vi "NewBooks.vi"(2 "Username":string="ME 184", 3 "Dialog?":enum16{"No Dialog", "Dialog", "Overwrite"}(ring)=enum."Dialog", 4 "Remote Path":string="bookfiles/") -> ()   [LabVIEW 2012]
uses:
  <vilib>/RoboBookEngine/Server/HTTPServer/Server2_Globals.vi
  <userlib>/BotSpeak/Devices/EvalRIO/FTPCodes/FTPParameters.ctl
panel:
  out "Prefix":string="ME184"
  in  "Parameters":T1={"Book Folder Name"="", "Full file name"="", "Remote Path"="bookfiles/", "Shelf folder"=path "", "Existing books"=[], "Dialog?"=enum."No Dialog", "New Format?"=FALSE}
  out "status":string
  in  "Close":bool
  in  "Download":bool
  in  "Books":i32[](listbox)
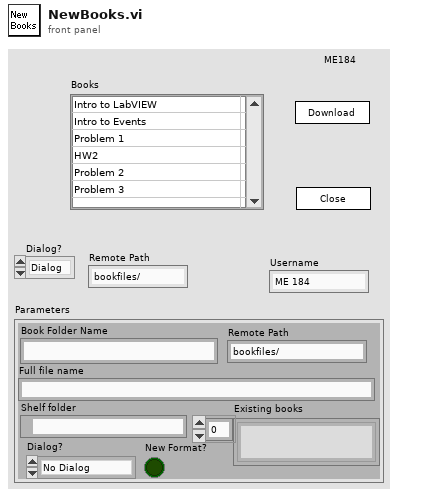
[diagram p1: front panel]
types:
  T1 = typedef "FTPParameters.ctl" = cluster{"Book Folder Name":string, "Full file name":string, "Remote Path":string, "Shelf folder":path, "Existing books":string[], "Dialog?":enum16{"No Dialog", "Dialog", "Overwrite"}, "New Format?":bool}
  T2 = typedef "PathsGlobal.ctl" = cluster{"Root":path, "Shelves":path, "Cmds":path, "Plugins":path}
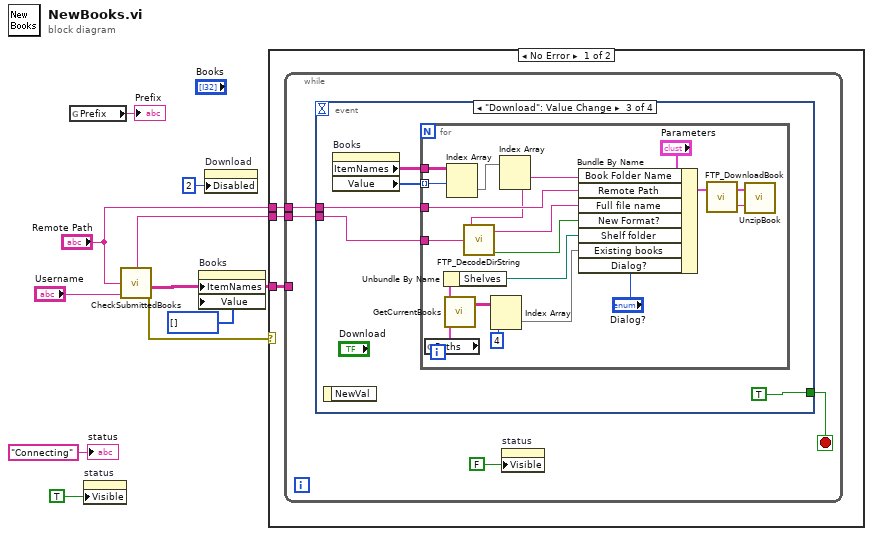
[diagram p0: block diagram]
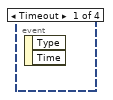
[diagram p2: hidden frame]
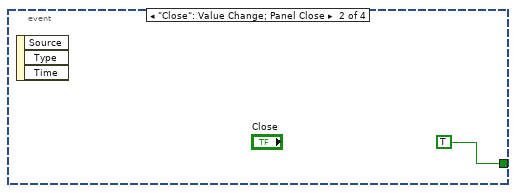
[diagram p3: hidden frame]
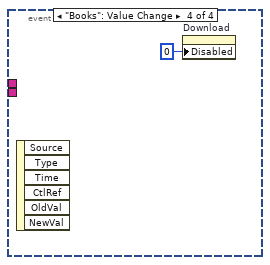
[diagram p4: hidden frame]
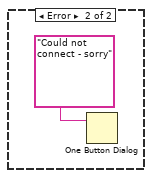
[diagram p5: hidden frame]
diagram:
  n1 = global read "Server2_Globals.vi" "Prefix"() -> (→"Prefix":string)
  n2 = property on="status" class="Str"("Visible"=TRUE) -> ()  [unwired: 2 in, 2 out]
  n3 = call <userlib>:"CheckSubmittedBooks.vi"("Username"="Username", "Remote Path"="Remote Path") -> ("error out"=w1:errorcluster, "submitted"=w5:string[][], "dropBox"=w4:string)  [unwired: 1 in, 3 out]
  n4 = property on="Books" class="MCListbox (strict)"("ItemNames"=w5, "Value"=i32[] [] ("Books")) -> ()  [unwired: 2 in, 2 out]
  n5 = property on="Download" class="Bool"("Disabled"=u8 2) -> ()  [unwired: 2 in, 2 out]
  n6 = case shown="No Error" w1 {
    tunnel: w5 -> [w13 _]
    tunnel: w4 -> [w12 _]
    tunnel: "Remote Path" -> [w11 _]
    frame No Error {
      n7 = while {
        tunnel: w13 -> [_]
        tunnel: w12 -> [w16]
        tunnel: w11 -> [w15]
        stop <- w17 stop-if-true
        n8 = event shown="[2] \"Download\": Value Change" {
          selector: _ -> [_ _ _ _]
          dyn-events: _ -> [_ _ _ _]
          timeout: _ -> [_ _ _ _]
          tunnel: [_ TRUE ("Close") TRUE ("Close") _] -> w17
          tunnel: w16 -> [_ _ w20 _]
          tunnel: w15 -> [_ _ w19 _]
          event Timeout {
            n9 = event-data() -> ()  [unwired: 3 out]
          }
          event "Close": Value Change; Panel Close {
            n10 = event-data() -> ()  [unwired: 4 out]
          }
          event "Download": Value Change {
            n11 = event-data() -> ()  [unwired: 2 out]
            n12 = property on="Books" class="MCListbox (strict)"() -> ("ItemNames"=w22:string[][], "Value"=w23:i32[])  [unwired: 2 in, 2 out]
            n13 = for {
              tunnel: w23 -> [w42] mode=indexing
              tunnel: w22 -> [w41]
              tunnel: w20 -> [w40]
              tunnel: w19 -> [w36]
              n14 = global read "Server2_Globals.vi" "Paths"() -> (w33:T2)
              n15 = Unbundle By Name(w33) -> ("Shelves"=w32:path)
              n16 = call <vilib>:"GetCurrentBooks.vi"("Paths"=w33) -> ("books"=w34:string[][])  [unwired: 2 in, 1 out]
              n17 = Index Array(array=w41, index (row)=w42) -> (element=w37:string[])  [unwired: 1 in]
              n18 = Index Array(array=w34, index (col)=4 ("disabled index (col)")) -> (element=w31:string[])  [unwired: 1 in]
              n19 = Index Array(array=w37) -> (element #1=w27:string, element #2=w24:string)  [unwired: 2 in]
              n20 = call <userlib>:"FTP_DecodeDirString.vi"("directory"=w40, "name"=w24) -> ("New Format?"=w26:bool, "Folder name"=w25:string)  [unwired: 4 out]
              n21 = Bundle By Name(cluster="Parameters", "Book Folder Name"=w27, "Remote Path"=w36, "Full file name"=w25, "New Format?"=w26, "Shelf folder"=w32, "Existing books"=w31, "Dialog?"="Dialog?") -> (w38:T1)
              n22 = call <userlib>:"FTP_DownloadBook.vi"("Parameters"=w38) -> ("ZipFile"=w29:string, "Parameters"=w30:T1)  [unwired: 1 in]
              n23 = call <userlib>:"UnzipBook.vi"("FileZipped"=w29, "Parameters"=w30) -> ()  [unwired: 1 in, 2 out]
            }
          }
          event "Books": Value Change {
            n24 = event-data() -> ()  [unwired: 7 out]
            n25 = property on="Download" class="Bool"("Disabled"=u8 0) -> ()  [unwired: 2 in, 2 out]
          }
        }
        n26 = property on="status" class="Str"("Visible"=FALSE) -> ()  [unwired: 2 in, 2 out]
      }
    }
    frame Error {
      n27 = One Button Dialog(message="Could not connect - sorry") -> ()  [unwired: 2 out]
    }
  }
  "status" <- "Connecting" ("status")
